vi "Ambient Conditions.vi"() -> ()   [LabVIEW 2017]
panel:
  out "Ambient Pressure":dbl format="%.2g"
  out "Ambient Temperature":dbl format="%.1g"
  in  "stop":bool
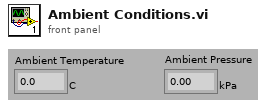
[diagram p1: front panel]
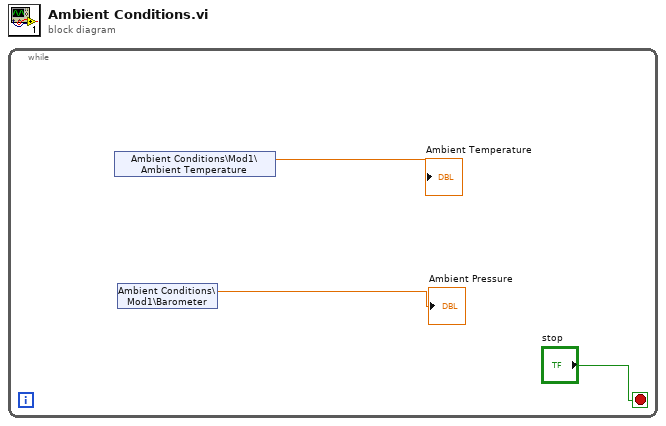
[diagram p0: block diagram]
diagram:
  n1 = while {
    stop <- "stop" stop-if-true
    n2 = shared-variable "Ambient Conditions\\Mod1\\Ambient Temperature"() -> (→"Ambient Temperature":dbl)  [unwired: 1 in, 1 out]
    n3 = shared-variable "Ambient Conditions\\Mod1\\Barometer"() -> (→"Ambient Pressure":dbl)  [unwired: 1 in, 1 out]
  }
